vi "SDG60SelectArbitraryWFM.vi"(7 "Channel (1:Channel 1)":i32(ring)=1 items=["Channel 1"=1, "Channel 2"=2], 8 "error in (no error)":errorcluster, 10 "WFM type (0:Builtin)":u16(ring)=1 items=["Builtin", "User"], 11 "VISA resource name":refnum<visa-resource-name>="USB0::0xF4EC::0x1101::SDG6XEBC5R0119::INSTR") -> (0 "error out":errorcluster, 3 "VISA resource name out":refnum<visa-resource-name>)   [LabVIEW 2018]
doc: "Selects an arbitrary waveform to output from the memory. Choose from built-in or user-defined arbitrary waveforms."
panel:
  in  "User WFM Number (ARB1)":i32=2
  in  "Waveform (0: Sine)":u16(ring) items=["Sine"=0, "Square"=47, "Pulse"=5, "Ramp"=8, "Noise"=1, "Triangle"=36]
  # "User WFM must be uploaded first. Must be followed by SDG60ConfArbWaveform1 \nThis can take ~8 s if large waveform\nGenerator doesn't show signs of being selected\nwhile this vi has already finished, but does eventually select."
  # "PRBS and DC are not builtin ARB functions\nUse STD waveform vi to select those"
  # "Possible indices 0-47. sine and noise don't work and are ignored by gnerator"
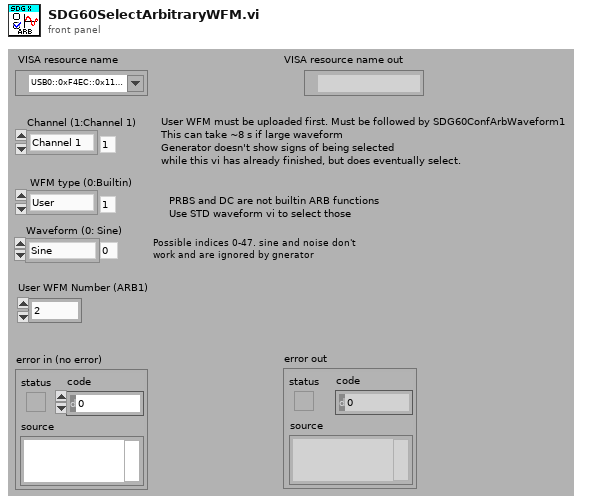
[diagram p1: front panel]
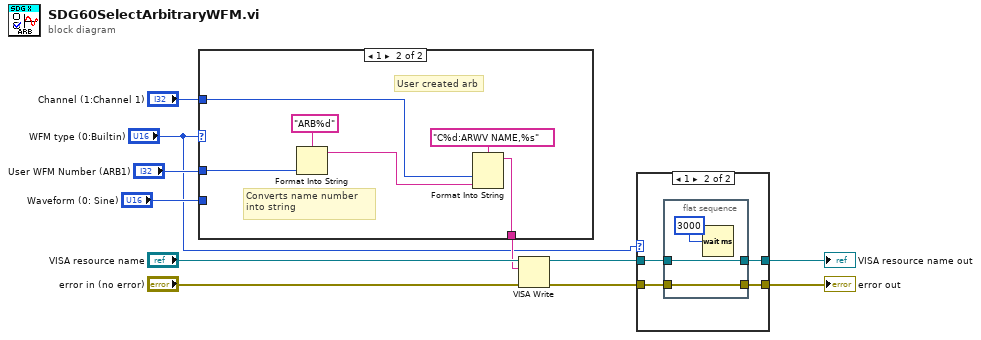
[diagram p0: block diagram]
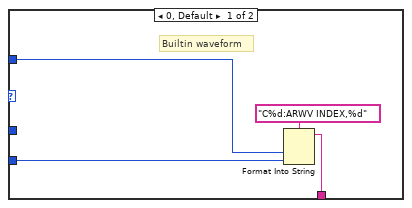
[diagram p3: hidden frame]
diagram:
  n1 = case shown="1" "WFM type (0:Builtin)" {
    tunnel: "Channel (1:Channel 1)" -> [w14 w21]
    tunnel: [w13 w19] -> w9
    tunnel: "User WFM Number (ARB1)" -> [_ w16]
    tunnel: "Waveform (0: Sine)" -> [w12 _]
    frame 0, Default {
      # "Builtin waveform"
      n2 = Format Into String(format string="C%d:ARWV INDEX,%d", w14, w12) -> (resulting string=w13:string)  [unwired: 2 in, 1 out]
    }
    frame 1 {
      # "Converts name number \ninto string"
      # "User created arb"
      n3 = Format Into String(format string="ARB%d", w16) -> (resulting string=w17:string)  [unwired: 2 in, 1 out]
      n4 = Format Into String(format string="C%d:ARWV NAME,%s", w21, w17) -> (resulting string=w19:string)  [unwired: 2 in, 1 out]
    }
  }
  n5 = VISA Write(VISA resource name="VISA resource name", write buffer=w9, error in (no error)="error in (no error)") -> (VISA resource name out=w7:refnum<visa-resource-name>, error out=w6:errorcluster)  [unwired: 1 out]
  n6 = case shown="1" "WFM type (0:Builtin)" {
    tunnel: w7 -> [w23 w27]
    tunnel: w6 -> [w22 w26]
    tunnel: [w22 w25] -> w5
    tunnel: [w23 w24] -> w4
    frame 0, Default {
      # "Delay only for\nuser wfms"
    }
    frame 1 {
      n7 = flat-sequence {
        tunnel: [w30] -> w24
        tunnel: w27 -> [w30]
        tunnel: w26 -> [w29]
        tunnel: [w29] -> w25
        frame #0 {
          n8 = Wait (ms)(milliseconds to wait=u32 3000 ("Delay Time (10)")) -> ()  [unwired: 1 out]
        }
      }
    }
  }
  "error out" <- w5
  "VISA resource name out" <- w4
